vi "Maxi Gauge-Parameter Control.vi"(6 "Set to default":i8(ring) items=["no change", "On"], 7 "W/R":bool, 8 "Fehler (Eingang)":errorcluster, 9 "Parameter lock":i8(ring)=2 items=["Off", "On", "no change"], 10 "Node address":i8=-1 min=-1 max=31 step=1, 11 "VISA-Ressource in":refnum<visa-resource-name>) -> (0 "Fehler (Ausgang)":errorcluster, 1 "Parameter lock Get":i8(ring) items=["Off", "On"], 3 "VISA-Ressource out":refnum<visa-resource-name>)   [LabVIEW 2013, in "Maxi Gauge.lvlib"]
uses:
  <instrlib>/Maxi Gauge/Maxi Gauge.lvlib
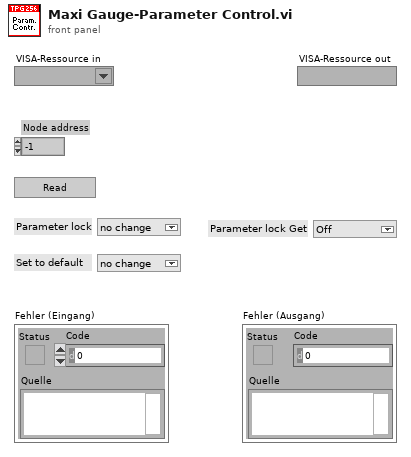
[diagram p1: front panel]
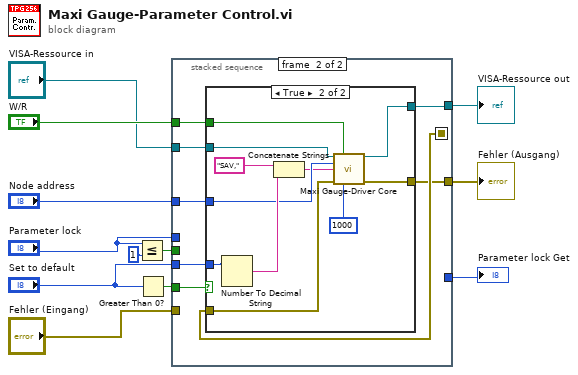
[diagram p0: block diagram]
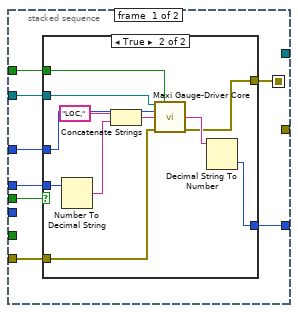
[diagram p2: hidden frame]
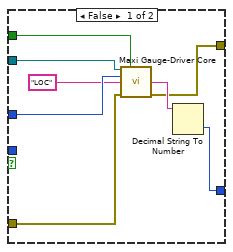
[diagram p3: hidden frame]
diagram:
  n1 = Less Or Equal?(x="Parameter lock", y=i8 1) -> (x <= y?=w6:bool)
  n2 = Greater Than 0?(x="Set to default") -> (x > 0?=w5:bool)
  n3 = stacked-sequence {
    seq-local: [w13 _] -> [_ w42]
    tunnel: "W/R" -> [w20 w47]
    tunnel: [w19 _] -> w8
    tunnel: "Parameter lock" -> [w18 _]
    tunnel: w5 -> [_ w46]
    tunnel: "Set to default" -> [_ w45]
    tunnel: "Node address" -> [w17 w44]
    tunnel: w6 -> [w16 _]
    tunnel: "Fehler (Eingang)" -> [w15 _]
    tunnel: "VISA-Ressource in" -> [w14 w43]
    tunnel: [_ w41] -> w2
    tunnel: [_ w40] -> w1
    frame #0 {
      n4 = case shown="True" w16 {
        tunnel: w20 -> [w27 w38]
        tunnel: [w26 w35] -> w19
        tunnel: w18 -> [_ w34]
        tunnel: [w25 w33] -> w13
        tunnel: w17 -> [w23 w32]
        tunnel: w15 -> [w24 w30]
        tunnel: w14 -> [w21 w29]
        frame False {
          n5 = call <instrlib>:"Maxi Gauge-Driver Core.vi"("VISA-Ressource in"=w21, "Write/Read"=w27, "Node address"=w23, "Command"="LOC", "Fehler (Eingang)"=w24) -> ("String Out"=w28:string, "Fehler (Ausgang)"=w25:errorcluster)  [unwired: 8 in, 1 out]
          n6 = Decimal String To Number(string=w28) -> (number=w26:i32)  [unwired: 2 in, 1 out]
        }
        frame True {
          n7 = Number To Decimal String(number=w34) -> (decimal integer string=w37:string)  [unwired: 1 in]
          n8 = Concatenate Strings("LOC,", w37) -> (w31:string)
          n9 = call <instrlib>:"Maxi Gauge-Driver Core.vi"("VISA-Ressource in"=w29, "Write/Read"=w38, "Node address"=w32, "Command"=w31, "Fehler (Eingang)"=w30) -> ("String Out"=w39:string, "Fehler (Ausgang)"=w33:errorcluster)  [unwired: 8 in, 1 out]
          n10 = Decimal String To Number(string=w39) -> (number=w35:i32)  [unwired: 2 in, 1 out]
        }
      }
    }
    frame #1 {
      n11 = case shown="True" w46 {
        tunnel: w47 -> [_ w60]
        tunnel: w45 -> [_ w57]
        tunnel: [w48 w56] -> w41
        tunnel: w44 -> [_ w54]
        tunnel: w42 -> [w48 w52]
        tunnel: w43 -> [w49 w51]
        tunnel: [w49 w50] -> w40
        frame False {
        }
        frame True {
          n12 = Number To Decimal String(number=w57) -> (decimal integer string=w59:string)  [unwired: 1 in]
          n13 = Concatenate Strings("SAV,", w59) -> (w53:string)
          n14 = call <instrlib>:"Maxi Gauge-Driver Core.vi"("VISA-Ressource in"=w51, "Write/Read"=w60, "Node address"=w54, "Command"=w53, "Fehler (Eingang)"=w52, "Timeout [ms]"=u32 1000) -> ("VISA-Ressource out"=w50:refnum<visa-resource-name>, "Fehler (Ausgang)"=w56:errorcluster)  [unwired: 7 in, 1 out]
        }
      }
    }
  }
  "Parameter lock Get" <- w8
  "Fehler (Ausgang)" <- w2
  "VISA-Ressource out" <- w1
